vi "Push.vi"(3 "Error In":errorcluster, 4 "Data":variant, 5 "object in":refnum<class "Stack.lvclass">) -> (0 "Error Out":errorcluster, 2 "object out":refnum<class "Stack.lvclass">)   [LabVIEW 2024, in "Stack.lvclass"]
doc: "24.1.1f1"
uses:
  Stack.lvclass
  Stack.lvclass/Stack.ctl
panel:
  # "Connector Pane"
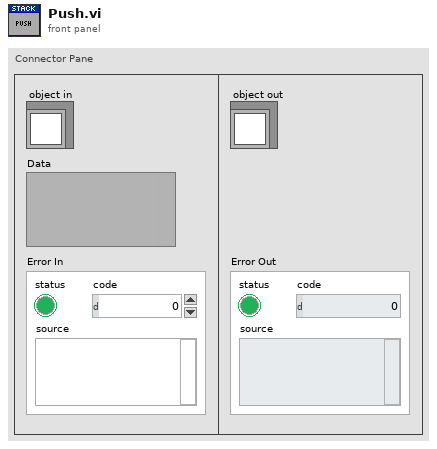
[diagram p1: front panel]
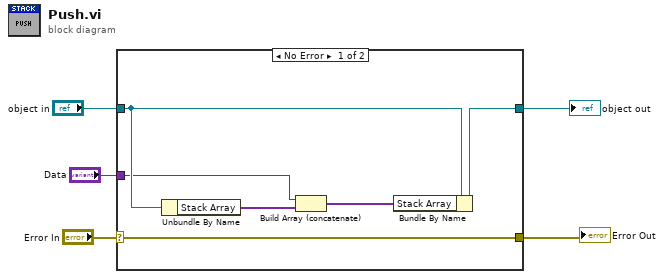
[diagram p0: block diagram]
diagram:
  n1 = case shown="No Error" "Error In" {
    selector: "Error In" -> [w11 w13]
    tunnel: [w11 w13] -> w4
    tunnel: [w9 w12] -> w2
    tunnel: "object in" -> [w10 w12]
    tunnel: "Data" -> [w6 _]
    frame No Error {
      n2 = Unbundle By Name(w10) -> ("Stack Array"=w7:variant[])
      n3 = Build Array (concatenate)(w6, w7) -> (w8:variant[])
      n4 = Bundle By Name(cluster=w10, "Stack Array"=w8) -> (w9:refnum<class "Stack.lvclass">)
    }
    frame Error {
    }
  }
  "Error Out" <- w4
  "object out" <- w2
